vi "InputTester.vi"() -> ()   [LabVIEW 2013]
uses:
  <vilib>/rvi/eio/common/nirviEmuTemplateMethod_errors.vi
  <vilib>/eio/EIONode/EIONode.xnode
panel:
  out "appended array":bool[](array[boolean])
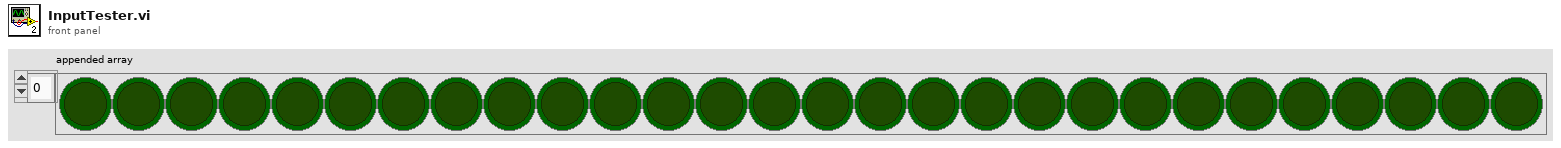
[diagram p1: front panel]
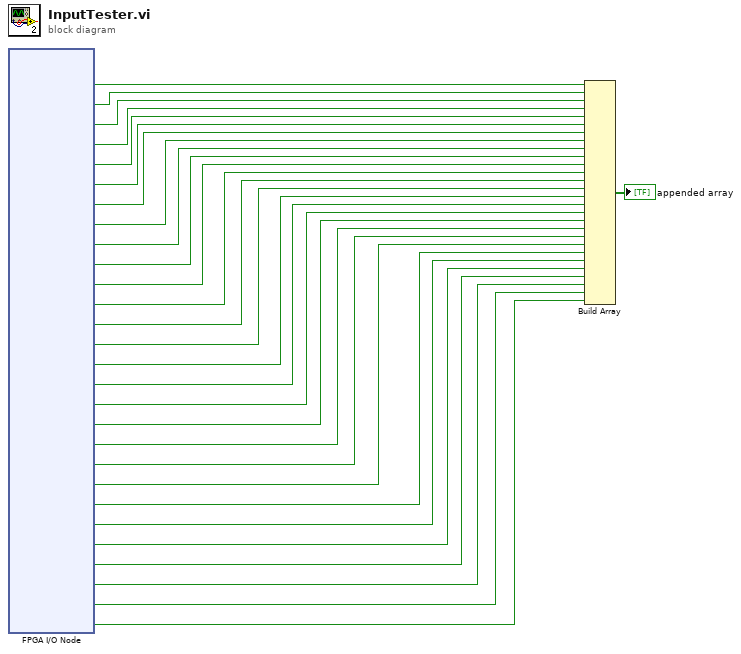
[diagram p0: block diagram]
diagram:
  n1 = xnode "FPGA I/O Node"() -> ("DIO0"=w29:bool, "DIO1"=w28:bool, "DIO2"=w27:bool, "DIO3"=w26:bool, "DIO4"=w25:bool, "DIO5"=w24:bool, "DIO6"=w23:bool, "DIO7"=w22:bool, "DIO8"=w21:bool, "DIO9"=w20:bool, "DIO10"=w19:bool, "DIO11"=w18:bool, "DIO12"=w17:bool, "DIO13"=w16:bool, "DIO14"=w15:bool, "DIO15"=w14:bool, "DIO16"=w13:bool, "DIO17"=w12:bool, "DIO18"=w11:bool, "DIO19"=w10:bool, "DIO20"=w9:bool, "DIO21"=w8:bool, "DIO22"=w7:bool, "DIO23"=w6:bool, "DIO24"=w5:bool, "DIO25"=w4:bool, "DIO26"=w3:bool, "DIO27"=w2:bool)  [unwired: 28 in, 28 out]
  n2 = Build Array(w29, w28, w27, w26, w25, w24, w23, w22, w21, w20, w19, w18, w17, w16, w15, w14, w13, w12, w11, w10, w9, w8, w7, w6, w5, w4, w3, w2) -> (→"appended array":bool[])
